vi "timer_sub_VI.vi"(10 "Reset":bool) -> (2 "Time (Secs)":dbl)   [LabVIEW 2016]
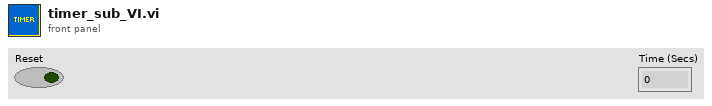
[diagram p1: front panel]
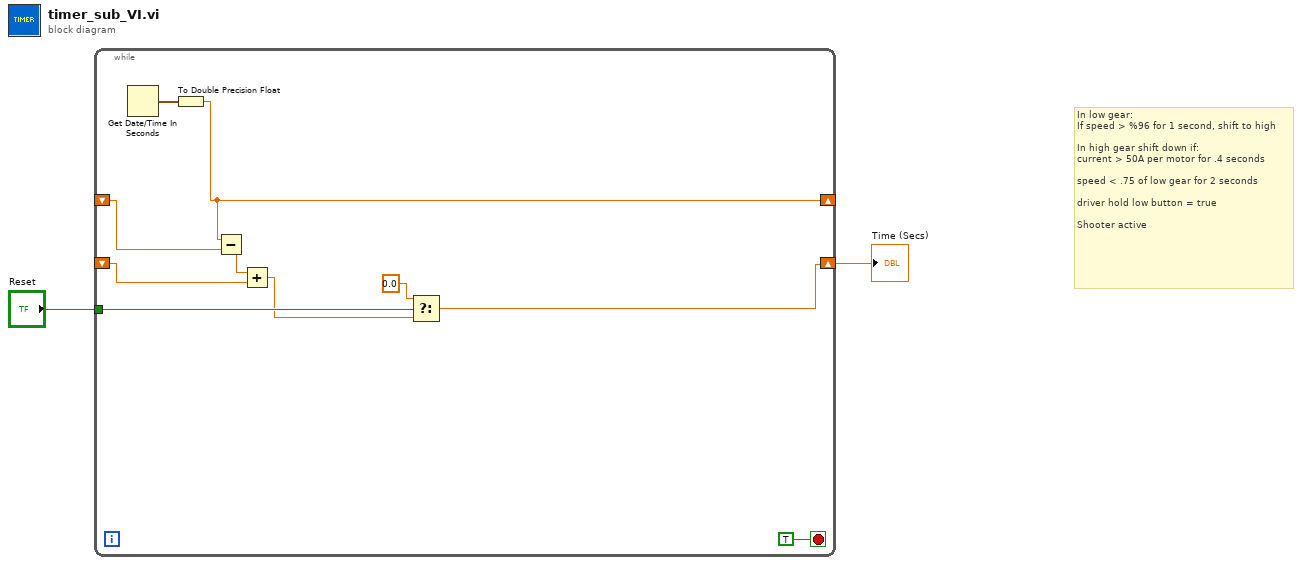
[diagram p0: block diagram]
diagram:
  # "In low gear:\nIf speed > %96 for 1 second, shift to high\n\nIn high gear shift down if:\ncurrent > 50A per motor for .4 seconds\n\nspeed < .75 of low gear for 2 seconds\n\ndriver hold low button = true\n\nShooter active"
  n1 = while {
    shift-right: [w10] -> _
    shift-left: _ -> [w11]
    shift-right: [w3] -> w2
    shift-left: _ -> [w8]
    tunnel: "Reset" -> [w6]
    stop <- TRUE stop-if-true
    n2 = Get Date/Time In Seconds() -> (seconds since 1Jan1904=w12:timestamp)
    n3 = To Double Precision Float(number=w12) -> (double precision float=w10:dbl)
    n4 = Subtract(x=w10, y=w11) -> (x-y=w9:dbl)
    n5 = Add(x=w9, y=w8) -> (x+y=w4:dbl)
    n6 = Select(t=0.0, s=w6, f=w4) -> (s? t:f=w3:dbl)
  }
  "Time (Secs)" <- w2
